vi "Interlock Chain Query.vi"(8 "error in (no error)":errorcluster, 11 "CO2 Actor in":refnum<class "CO2 Actor.lvclass">) -> (0 "error out":errorcluster, 1 "Interlock out":bool, 3 "CO2 Actor out":refnum<class "CO2 Actor.lvclass">, 4 "Stop Self?":bool)   [LabVIEW 2015, in "cRIO-Carbondioxide.lvlib" / "CO2-Actor.lvlib" / "CO2 Actor.lvclass"]
uses:
  CO2 Actor.lvclass
  CO2 Actor.lvclass/CO2 Actor.ctl
  <vilib>/ActorFramework/Actor/Actor.lvclass/Actor.ctl
  <vilib>/ActorFramework/Message Enqueuer/Message Enqueuer.lvclass/Message Enqueuer.ctl
  Interlocks/Interlock/Interlock.lvclass/Interlock.ctl
  <vilib>/ActorFramework/Actor/Read Self Enqueuer.vi
  <vilib>/ActorFramework/Message Enqueuer/Init from Existing Queue.vi
  <vilib>/ActorFramework/Message Enqueuer/Message Enqueuer.lvclass
  <vilib>/ActorFramework/Actor/Actor.lvclass
  Interlocks/Interlock Chain/Interlock Chain.lvclass
  Interlocks/Interlock/Interlock.lvclass
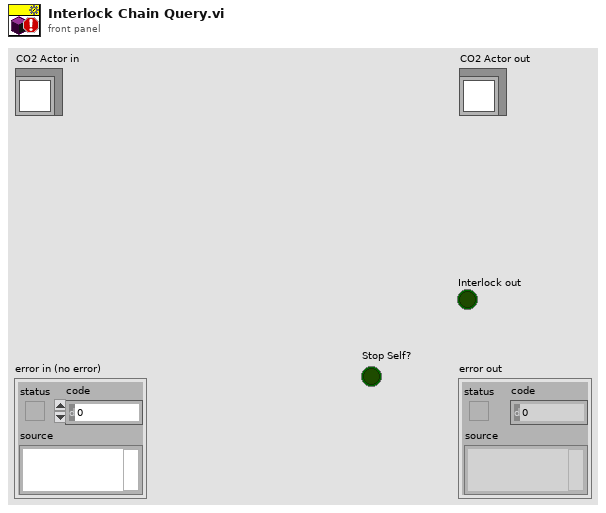
[diagram p1: front panel]
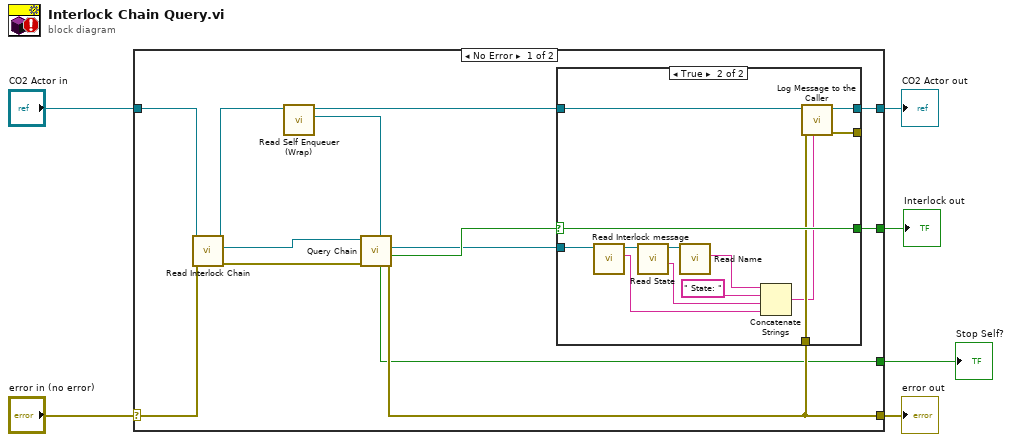
[diagram p0: block diagram]
diagram:
  n1 = case shown="No Error" "error in (no error)" {
    selector: "error in (no error)" -> [w18 w36]
    tunnel: [w12 w36] -> w5
    tunnel: [w11 w35] -> w3
    tunnel: "CO2 Actor in" -> [w17 w35]
    tunnel: [w16 _] -> w2
    tunnel: [w7 _] -> w1
    frame No Error {
      n2 = call "Read Interlock Chain.vi"("error in (no error)"=w18, "CO2 Actor in"=w17) -> ("error out"=w15:errorcluster, "Interlock Chain"=w19:refnum<class "Interlock Chain.lvclass">, "CO2 Actor out"=w10:refnum<class "CO2 Actor.lvclass">)  [unwired: 7 in]
      n3 = call "Read Self Enqueuer (Wrap).vi"("CO2 Actor in"=w10) -> ("Actor Framework:Message Enqueuer"=w9:refnum<class "Message Enqueuer.lvclass">, "CO2 Actor out"=w8:refnum<class "CO2 Actor.lvclass">)  [unwired: 9 in]
      n4 = call "Query Chain.vi"("Caller Enqueuer"=w9, "error in (no error)"=w15, "Interlock Chain"=w19) -> ("error out"=w12:errorcluster, "Interlock?"=w14:bool, "Interlock out"=w13:refnum<class "Interlock.lvclass">, "Stop Self?"=w7:bool)  [unwired: 3 in, 2 out]
      n5 = case shown="True" w14 {
        selector: w14 -> [w21 w34]
        tunnel: w13 -> [_ w33]
        tunnel: [w21 w34] -> w16
        tunnel: w12 -> [_ w24]
        tunnel: w8 -> [w20 w26]
        tunnel: [w20 w25] -> w11
        tunnel: [_ w23] -> _
        frame False {
        }
        frame True {
          n6 = call "Read Interlock message.vi"("Interlock in"=w33) -> ("Interlock message"=w27:string, "Interlock out"=w28:refnum<class "Interlock.lvclass">)  [unwired: 9 in]
          n7 = call "Read State.vi"("Interlock in"=w28) -> ("State string"=w30:string, "Interlock out"=w32:refnum<class "Interlock.lvclass">)  [unwired: 8 in, 1 out]
          n8 = call "Read Name.vi"("Interlock in"=w32) -> ("Name"=w29:string)  [unwired: 9 in, 1 out]
          n9 = Concatenate Strings(w29, " State: " ("string"), w30, w27) -> (w22:string)
          n10 = call-dynamic "Log Message to the Caller.vi"("String (\"\" = no message to send)"=w22, "error in (no error)"=w24, "CO2 Actor in"=w26) -> ("error out"=w23:errorcluster, "CO2 Actor out"=w25:refnum<class "CO2 Actor.lvclass">)  [unwired: 7 in]
        }
      }
    }
    frame Error {
    }
  }
  "error out" <- w5
  "CO2 Actor out" <- w3
  "Interlock out" <- w2
  "Stop Self?" <- w1
